vi "Read Enabled Channels.vi"(8 "error in (no error)":errorcluster, 11 "Multi Parser in":refnum<class "Mulit Sentence Parser.lvclass">) -> (0 "error out":errorcluster, 2 "Enabled Channels":string[](array[string]), 3 "Multi Parser out":refnum<class "Mulit Sentence Parser.lvclass">)   [LabVIEW 2018, in "Mulit Sentence Parser.lvclass"]
doc: "Multi Sentence Parser.lvclass:Read Enabled Channels.vi\n\nThis VI returns the list of channel names that are enabled for the Multi Sentence Parser class.\n\nInstrument Communication Module Version 1.0\nOctober, 2018 Original Code Consulting David Thomson\n www.originalcode.com"
uses:
  Mulit Sentence Parser.lvclass
  Mulit Sentence Parser.lvclass/Mulit Sentence Parser.ctl
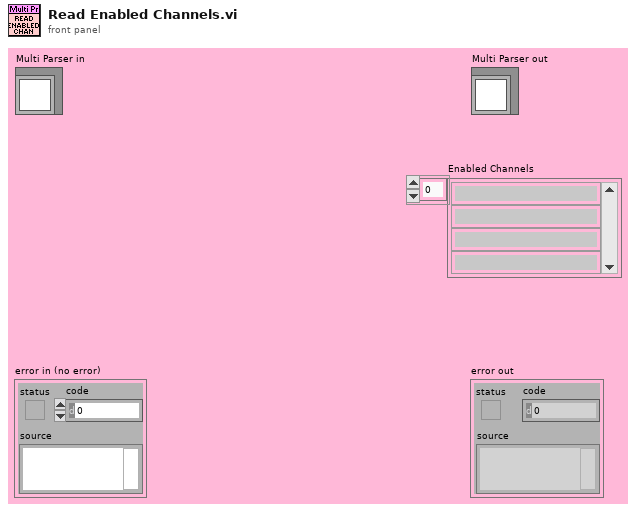
[diagram p1: front panel]
types:
  T1 = cluster{"Sentence ID":string, "Format String":string, "Channels":string[], "Enabled":bool[]}[]
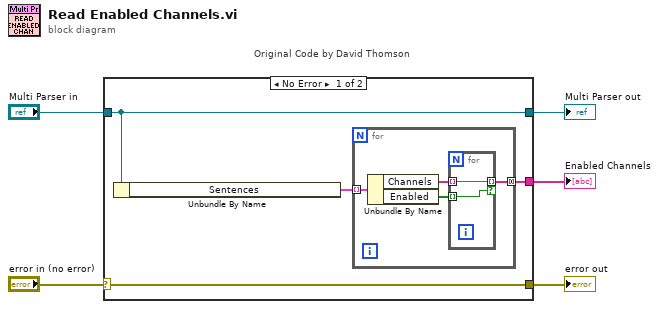
[diagram p0: block diagram]
diagram:
  n1 = case "Original Code by David Thomson" shown="No Error" "error in (no error)" {
    selector: "error in (no error)" -> [w9 w16]
    tunnel: [w9 w16] -> w4
    tunnel: [w7 w17] -> w2
    tunnel: "Multi Parser in" -> [w7 w17]
    tunnel: [w8 _] -> w1
    frame No Error {
      n2 = Unbundle By Name(w7) -> ("Sentences"=w6:T1)
      n3 = for {
        tunnel: [w11] -> w8 mode=concatenating
        tunnel: w6 -> [w10] mode=indexing
        n4 = Unbundle By Name(w10) -> ("Channels"=w13:string[], "Enabled"=w12:bool[])
        n5 = for {
          tunnel: [w15] -> w11 mode=indexing if=w14
          tunnel: w13 -> [w15] mode=indexing
          tunnel: w12 -> [w14] mode=indexing
        }
      }
    }
    frame Error {
    }
  }
  "error out" <- w4
  "Multi Parser out" <- w2
  "Enabled Channels" <- w1
